vi "CPU_MEM_kernal_ROM.vi"(4 "read all":bool, 5 "init size":u16=8191 format="%.0x", 7 "oper":enum16{"init", "read", "write"}(ring), 10 "value in":u8 format="%02x", 11 "address":u16 format="%04x") -> (2 "value out":u8 format="%02x", 3 "mem":u8[](array[numeric]))   [LabVIEW 2018]
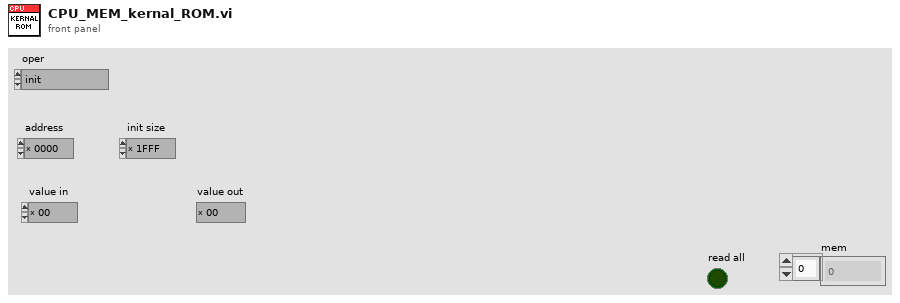
[diagram p1: front panel]
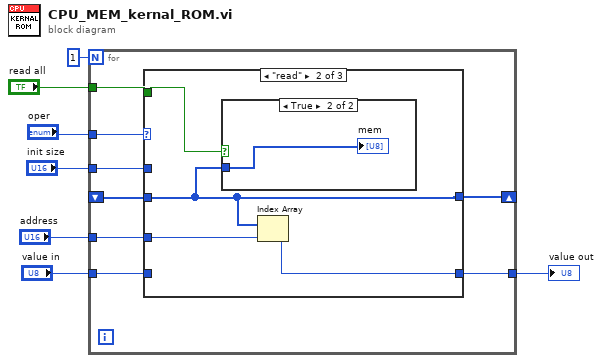
[diagram p0: block diagram]
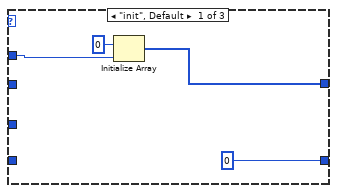
[diagram p2: hidden frame]
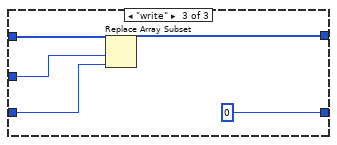
[diagram p4: hidden frame]
diagram:
  n1 = for {
    N: 1 -> [_]
    shift-right: [w13] -> _
    shift-left: _ -> [w12]
    tunnel: "oper" -> [w15]
    tunnel: "init size" -> [w14]
    tunnel: [w11] -> w4
    tunnel: "address" -> [w10]
    tunnel: "value in" -> [w9]
    tunnel: "read all" -> [w8]
    n2 = case shown="\"read\"" w15 {
      tunnel: w14 -> [w16 _ _]
      tunnel: [w18 w21 w26] -> w13
      tunnel: w12 -> [_ w21 w29]
      tunnel: [u8 0 ("element") w23 u8 0 ("element")] -> w11
      tunnel: w10 -> [_ w22 w28]
      tunnel: w9 -> [_ _ w27]
      tunnel: w8 -> [_ w20 _]
      frame "init", Default {
        n3 = Initialize Array(u8 0 ("element"), w16) -> (w18:u8[])
      }
      frame "read" {
        n4 = case shown="True" w20 {
          tunnel: w21 -> [_ w24]
          frame False {
          }
          frame True {
            "mem" <- w24
          }
        }
        n5 = Index Array(array=w21, index=w22) -> (element=w23:u8)
      }
      frame "write" {
        n6 = Replace Array Subset(array=w29, new element=w27, index=w28) -> (w26:u8[])
      }
    }
  }
  "value out" <- w4
